vi "Create Metadata Response.vi"(8 "error in":errorcluster, 9 "gRPC ID":T9, 10 "measurement plugin service in":refnum<class "Measurement Plugin Service.lvclass">) -> (0 "error out":errorcluster, 2 "get metadata response":T1, 3 "gRPC ID out":T9)   [LabVIEW 2020, in "Measurement Plugin Measurement Server.lvlib" / "IMeasurement Service.lvclass"]
uses:
  IMeasurement Service.lvclass
  <vilib>/gRPC/LabVIEW gRPC Library/Shared/grpcId.ctl
  Helpers/TypeDefs/Get Metadata Response.ctl
  Helpers/TypeDefs/Measurement Details.ctl
  Helpers/TypeDefs/Measurement Signature.ctl
  Helpers/TypeDefs/Configuration Parameter.ctl
  Helpers/TypeDefs/Parameter Annotations Entry.ctl
  <vilib>/gRPC/LabVIEW gRPC Library/Shared/Any.ctl
  Helpers/TypeDefs/Output Parameter.ctl
  Helpers/TypeDefs/User Interface Details.ctl
  Measurement Plugin Service/Measurement Plugin Service.lvclass
  <vilib>/gRPC/LabVIEW gRPC Library/Server API/typeDefs/gRPC Status Code.ctl
  Measurement Plugin Measurement Server.lvlib
  <vilib>/gRPC/LabVIEW gRPC Library/grpc-lvsupport-release.lvlib
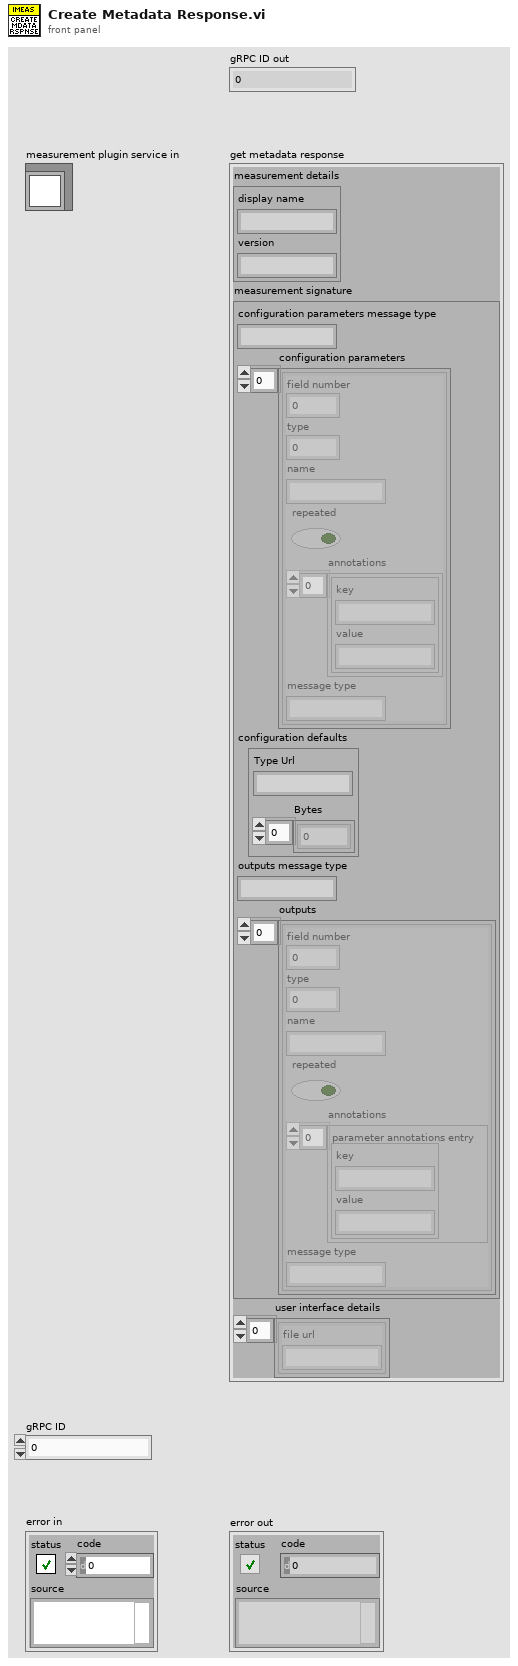
[diagram p1: front panel]
types:
  T1 = typedef "Measurement Plugin Measurement Server.lvlib/Get Metadata Response.ctl" = cluster{"measurement details":T2, "measurement signature":T3, "user interface details":T8[]}
  T2 = typedef "Measurement Plugin Measurement Server.lvlib/Measurement Details.ctl" = cluster{"display name":string, "version":string}
  T3 = typedef "Measurement Plugin Measurement Server.lvlib/Measurement Signature.ctl" = cluster{"configuration parameters message type":string, "configuration parameters":T4[], "configuration defaults":T6, "outputs message type":string, "outputs":T7[]}
  T4 = typedef "Measurement Plugin Measurement Server.lvlib/Configuration Parameter.ctl" = cluster{"field number":i32, "type":i32, "name":string, "repeated":bool, "annotations":T5[], "message type":string}
  T5 = typedef "Measurement Plugin Measurement Server.lvlib/Parameter Annotations Entry.ctl" = cluster{"key":string, "value":string}
  T6 = typedef "grpc-lvsupport-release.lvlib/Any.ctl" = cluster{"Type Url":string, "Bytes":u8[]}
  T7 = typedef "Measurement Plugin Measurement Server.lvlib/Output Parameter.ctl" = cluster{"field number":i32, "type":i32, "name":string, "repeated":bool, "annotations":T5[], "message type":string}
  T8 = typedef "Measurement Plugin Measurement Server.lvlib/User Interface Details.ctl" = cluster{"file url":string}
  T9 = typedef "grpc-lvsupport-release.lvlib/grpcId.ctl" = u64
  T10 = typedef "grpc-lvsupport-release.lvlib/gRPC Status Code.ctl" = enum16{"OK", "CANCELLED", "UNKNOWN", "INVALID_ARGUMENT", "DEADLINE_EXCEEDED", "NOT_FOUND", "ALREADY_EXISTS", "PERMISSION_DENIED", "RESOURCE_EXHAUSTED", "FAILED_PRECONDITION", "ABORTED", "OUT_OF_RANGE", "UNIMPLEMENTED", "INTERNAL", "UNAVAILABLE", "DATA_LOSS", "UNAUTHENTICATED"}
  T11 = typedef "Measurement Plugin Measurement Server.lvlib/Measurement Plugin Service.lvclass/Plugin Paths.ctl" = cluster{"get measurement details VI path":path, "get type specializations VI path":path, "get UI details VI path":path, "measurement logic VI path":path, "measurement configuration ctl path":path, "measurement results ctl path":path}
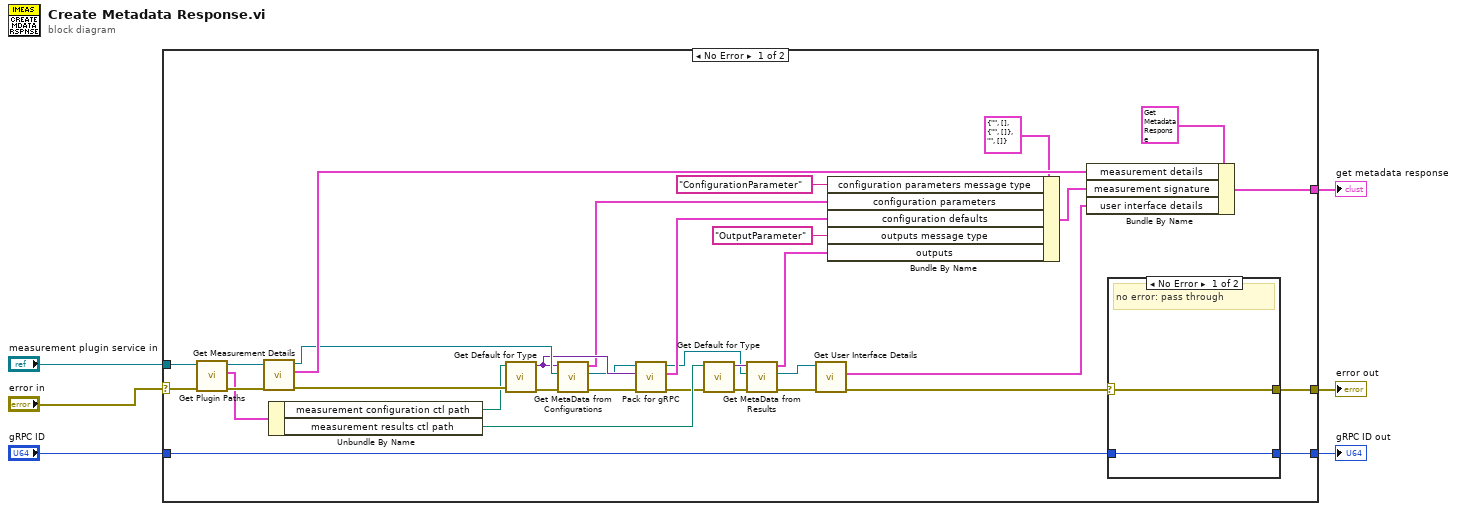
[diagram p0: block diagram]
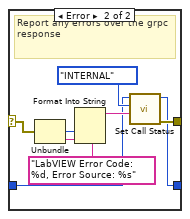
[diagram p2: hidden frame]
diagram:
  n1 = case shown="No Error" "error in" {
    selector: "error in" -> [w10 w53]
    tunnel: [w35 w52] -> w6
    tunnel: "gRPC ID" -> [w34 w52]
    tunnel: [w33 w53] -> w4
    tunnel: [w31 _] -> w3
    tunnel: "measurement plugin service in" -> [w27 _]
    frame No Error {
      n2 = call-dynamic "Get Plugin Paths.vi"("error in"=w10, "measurement plugin service in"=w27) -> ("error out"=w38:errorcluster, "plugin paths"=w28:T11, "measurement plugin service out"=w36:refnum<class "Measurement Plugin Service.lvclass">)  [unwired: 7 in]
      n3 = call-dynamic "Get Measurement Details.vi"("error in"=w38, "measurement plugin service in"=w36) -> ("error out"=w39:errorcluster, "measurement details"=w40:T2, "measurement plugin service out"=w37:refnum<class "Measurement Plugin Service.lvclass">)  [unwired: 5 in, 2 out]
      n4 = Unbundle By Name(w28) -> ("measurement configuration ctl path"=w29:path, "measurement results ctl path"=w30:path)
      n5 = call "Get Default for Type.vi"("error in"=w39, "path of type"=w29) -> ("error out"=w16:errorcluster, "default for type"=w23:variant)  [unwired: 8 in]
      n6 = call "Get MetaData from Configurations.vi"("error in"=w16, "measurement plugin service in"=w37, "configuration cluster"=w23) -> ("error out"=w22:errorcluster, "measurement plugin service out"=w8:refnum<class "Measurement Plugin Service.lvclass">, "configuration parameters"=w11:T4[])  [unwired: 6 in]
      n7 = call-dynamic "Pack for gRPC.vi"("error in"=w22, "data value"=w23, "measurement plugin service in"=w8) -> ("error out"=w25:errorcluster, "any"=w24:T6, "measurement plugin service out"=w9:refnum<class "Measurement Plugin Service.lvclass">)  [unwired: 6 in]
      n8 = call "Get Default for Type.vi"("error in"=w25, "path of type"=w30) -> ("error out"=w21:errorcluster, "default for type"=w20:variant)  [unwired: 8 in]
      n9 = call "Get MetaData from Results.vi"("error in"=w21, "measurement plugin service in"=w9, "results cluster"=w20) -> ("error out"=w15:errorcluster, "measurement plugin service out"=w7:refnum<class "Measurement Plugin Service.lvclass">, "outputs"=w12:T7[])  [unwired: 6 in]
      n10 = call-dynamic "Get User Interface Details.vi"("error in"=w15, "measurement plugin service in"=w7) -> ("error out"=w32:errorcluster, "user interface details"=w26:T8[])  [unwired: 7 in, 1 out]
      n11 = Bundle By Name(cluster=T3 {"configuration parameters message type"="", "configuration parameters"=[], "configuration defaults"={"Type Url"="", "Bytes"=[]}, "outputs message type"="", "outputs"=[]} ("ni_measurements_v1_MeasurementSignature"), "configuration parameters message type"="ConfigurationParameter" ("configuration_parameters_messagetype"), "configuration parameters"=w11, "configuration defaults"=w24, "outputs message type"="OutputParameter" ("configuration_parameters_messagetype"), "outputs"=w12) -> (w18:T3)
      n12 = Bundle By Name(cluster=T1 {"measurement details"={"display name"="", "version"=""}, "measurement signature"={"configuration parameters message type"="", "configuration parameters"=[], "configuration defaults"={"Type Url"="", "Bytes"=[]}, "outputs message type"="", "outputs"=[]}, "user interface details"=[]} ("package_templatemessage"), "measurement details"=w40, "measurement signature"=w18, "user interface details"=w26) -> (w31:T1)
      n13 = case shown="No Error" w32 {
        selector: w32 -> [w41 w45]
        tunnel: [w41 w46] -> w33
        tunnel: w34 -> [w42 w44]
        tunnel: [w42 w43] -> w35
        frame No Error {
          # "no error: pass through"
        }
        frame Error {
          # "Report any errors over the grpc response"
          n14 = Unbundle(w45) -> ("code"=w49:i32, "source"=w50:string)  [unwired: 1 out]
          n15 = Format Into String(format string="LabVIEW Error Code: %d, Error Source: %s", w49, w50) -> (resulting string=w51:string)  [unwired: 2 in, 1 out]
          n16 = call <vilib>:"Set Call Status.vi"("Details"=w51, "Status Code"=gRPC_Status_Code."INTERNAL", "gRPCid in"=w44) -> ("error out"=w46:errorcluster, "gRPCid out"=w43:T9)  [unwired: 7 in]
        }
      }
    }
    frame Error {
    }
  }
  "gRPC ID out" <- w6
  "error out" <- w4
  "get metadata response" <- w3
